vi "IMAQdx Start Acquisition.vi"(8 "error in":errorcluster, 11 "Session In":T1) -> (0 "error out":errorcluster, 3 "Session Out":T1)   [LabVIEW 2020, in "NI_Vision_Acquisition_Software.lvlib"]
doc: "Starts an acquisition that was previously configured with the IMAQdx Configure Acquisition VI. Use the IMAQdx Stop Acquisition VI to stop the acquisition."
uses:
  NI_Vision_Acquisition_Software.lvlib
  IMAQdx.ctl
  niimaqdx.dll
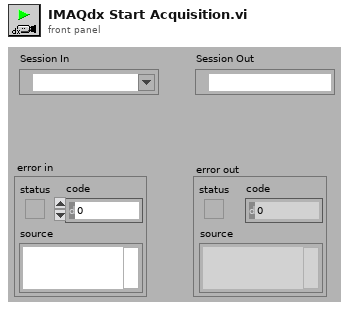
[diagram p1: front panel]
types:
  T1 = typedef "IMAQdx.ctl" = refnum<k21>
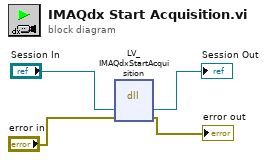
[diagram p0: block diagram]
diagram:
  n1 = dll-call lib="niimaqdx.dll" fn="LV_IMAQdxStartAcquisition"("Session In"="Session In", "error in"="error in") -> ("Session In"=→"Session Out":T1, "error in"=→"error out":errorcluster)  [unwired: 4 in, 2 out]
